vi "compatOpenFileOperation.vi"(1 "operation (existing)":T2(ring)=enum."new or existing, truncate") -> (0 "operation (open)":T1(ring))   [LabVIEW 2020]
doc: "Converts the old Open File Operation Enum to the new one."
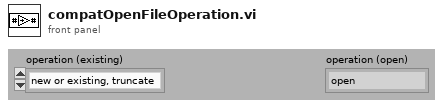
[diagram p1: front panel]
types:
  T1 = enum16{"open", "replace", "create", "open or create", "replace or create", "replace or create with confirmation"}
  T2 = enum16{"existing only", "existing only, truncate", "new only", "new or existing", "new or existing, truncate", "new or existing (confirm dialog)", "new or existing, truncate (confirm dialog)"}
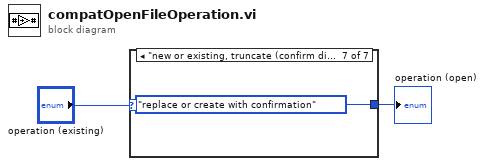
[diagram p0: block diagram]
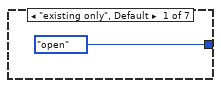
[diagram p2: hidden frame]
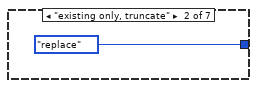
[diagram p3: hidden frame]
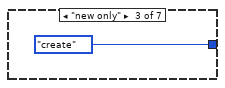
[diagram p4: hidden frame]
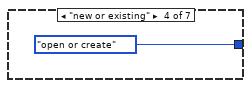
[diagram p5: hidden frame]
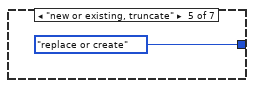
[diagram p6: hidden frame]
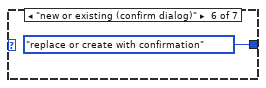
[diagram p7: hidden frame]
diagram:
  n1 = case shown="\"new or existing, truncate (confirm dialog)\"" "operation (existing)" {
    tunnel: [T1."open" ("operation (open)") T1."replace" ("operation (open)") T1."create" ("operation (open)") T1."open or create" ("operation (open)") T1."replace or create" ("operation (open)") T1."replace or create with confirmation" ("operation (open)") T1."replace or create with confirmation" ("operation (open)")] -> w1
    frame "existing only", Default {
    }
    frame "existing only, truncate" {
    }
    frame "new only" {
    }
    frame "new or existing" {
    }
    frame "new or existing, truncate" {
    }
    frame "new or existing (confirm dialog)" {
    }
    frame "new or existing, truncate (confirm dialog)" {
    }
  }
  "operation (open)" <- w1
